vi "Init Control Value - Num.vi"(8 "error in (no error)":errorcluster, 10 "Num Control Names":string[](array[string]), 11 "This VI":refnum<vi>) -> (0 "error out":errorcluster, 2 "PLC IP":string, 3 "Config File Path":path)   [LabVIEW 2018]
uses:
  <vilib>/Utility/config.llb/Read Key (Double).vi
  <vilib>/Utility/config.llb/Write Key (Double).vi
  <vilib>/Utility/config.llb/Read Key (String).vi
  <vilib>/Utility/config.llb/NI_LVConfig.lvlib
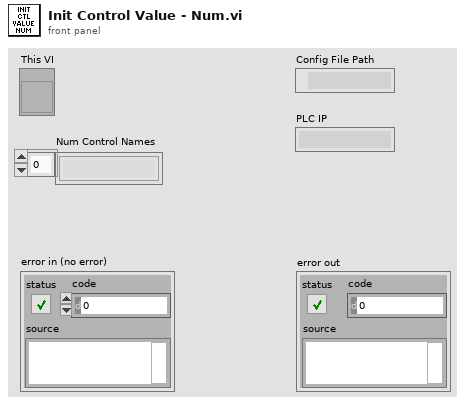
[diagram p1: front panel]
types:
  T1 = typedef "NI_LVConfig.lvlib/Config Data RefNum.ctl" = refnum<k1>
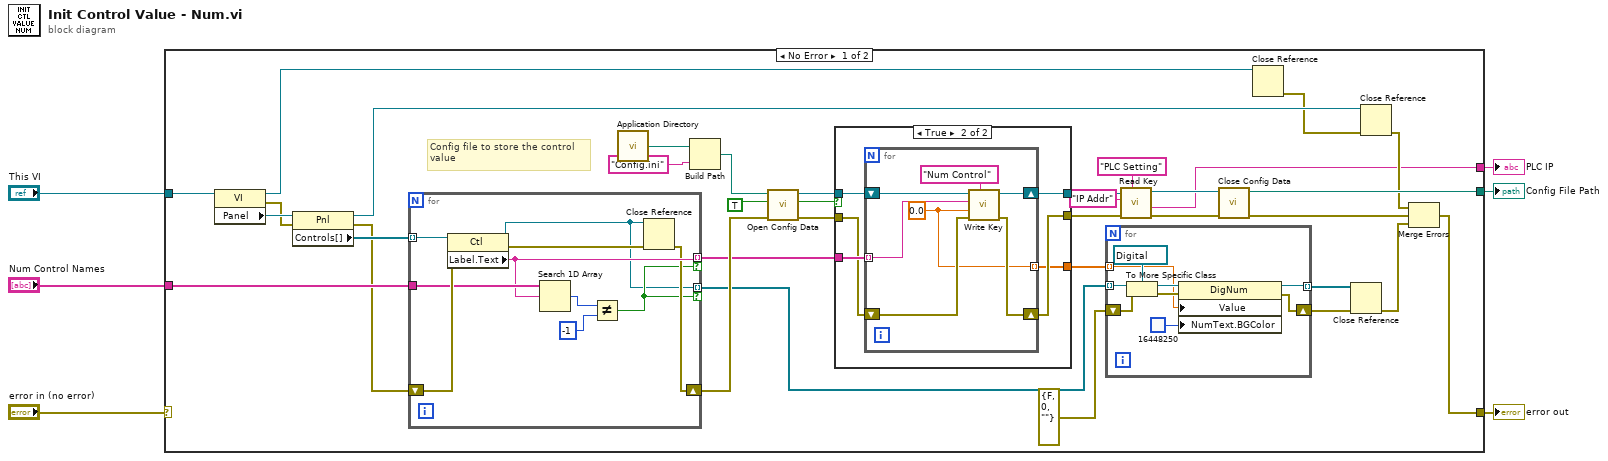
[diagram p0: block diagram]
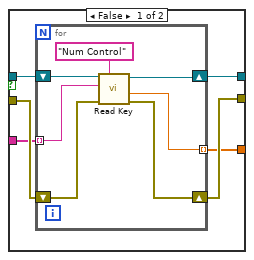
[diagram p2: hidden frame]
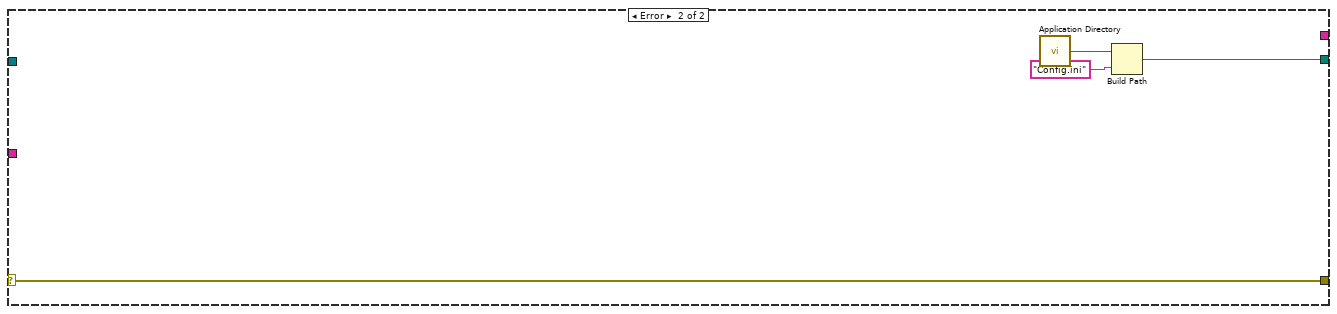
[diagram p3: hidden frame]
diagram:
  n1 = case shown="No Error" "error in (no error)" {
    selector: "error in (no error)" -> [_ w87]
    tunnel: "Num Control Names" -> [w38 _]
    tunnel: "This VI" -> [w39 _]
    tunnel: [w23 w88] -> w2
    tunnel: [w20 w87] -> w3
    tunnel: [w7 _] -> w1
    frame No Error {
      # "Config file to store the control\nvalue"
      n2 = property class="VI"(reference=w39) -> (reference out=w26:refnum<vi>, error out=w40:errorcluster, "Panel"=w41:refnum<vi>)  [unwired: 1 in]
      n3 = property class="Pnl"(reference=w41, error in=w40) -> (reference out=w25:refnum<vi>, error out=w36:errorcluster, "Controls[]"=w37:refnum<vi>[])
      n4 = for {
        tunnel: w37 -> [w86] mode=indexing
        shift-right: [w79] -> w34
        shift-left: w36 -> [w85]
        tunnel: w38 -> [w84]
        tunnel: [w81] -> w31 mode=indexing if=w78
        tunnel: [w77] -> w18 mode=indexing if=w78
        n5 = property class="Ctl"(reference=w86, error in=w85) -> (reference out=w77:refnum<vi>, error out=w80:errorcluster, "Label.Text"=w81:string)
        n6 = Search 1D Array(1D array=w84, element=w81) -> (index of element=w83:i32)  [unwired: 1 in]
        n7 = Not Equal?(x=w83, y=-1) -> (x != y?=w78:bool)
        n8 = Close Reference(reference=w77, error in (no error)=w80) -> (error out=w79:errorcluster)
      }
      n9 = call <vilib>:"Application Directory.vi"() -> ("Application Directory"=w29:path)
      n10 = Build Path(base path=w29, name or relative path="Config.ini") -> (appended path=w27:path)
      n11 = call <vilib>:"Open Config Data.vi"("error in (no error)"=w34, "create file if necessary (T)"=TRUE, "configuration file path"=w27) -> ("error out"=w30:errorcluster, "file created?"=w33:bool, "refnum"=w32:T1)  [unwired: 6 in]
      n12 = case shown="True" w33 {
        tunnel: w32 -> [w56 w68]
        tunnel: w31 -> [w54 w69]
        tunnel: w30 -> [w55 w67]
        tunnel: [w53 w66] -> w13
        tunnel: [w52 w65] -> w12
        tunnel: [w51 w64] -> w17
        frame False {
          n13 = for {
            shift-right: [w60] -> w53
            shift-left: w56 -> [w63]
            shift-right: [w58] -> w52
            shift-left: w55 -> [w61]
            tunnel: w54 -> [w59] mode=indexing
            tunnel: [w57] -> w51 mode=indexing
            n14 = call-poly <vilib>:"Read Key.vi"("section"="Num Control", "error in (no error)"=w61, "key"=w59, "refnum"=w63) -> ("error out"=w58:errorcluster, "value"=w57:dbl, "refnum out"=w60:T1)  [unwired: 4 in, 1 out]
          }
        }
        frame True {
          n15 = for {
            tunnel: w69 -> [w74] mode=indexing
            shift-right: [w72] -> w66
            shift-left: w68 -> [w75]
            shift-right: [w71] -> w65
            shift-left: w67 -> [w73]
            tunnel: [w70] -> w64 mode=indexing
            w70 = 0.0
            n16 = call-poly <vilib>:"Write Key.vi"("section"="Num Control", "error in (no error)"=w73, "value"=w70, "key"=w74, "refnum"=w75) -> ("error out"=w71:errorcluster, "refnum out"=w72:T1)  [unwired: 3 in, 2 out]
          }
        }
      }
      n17 = for {
        tunnel: w18 -> [w46] mode=indexing
        shift-right: [w43] -> w14
        shift-left: errorcluster {"status"=FALSE, "code"=0, "source"=""} ("error constant") -> [w45]
        tunnel: w17 -> [w44] mode=indexing
        tunnel: [w42] -> w16 mode=indexing
        n18 = To More Specific Class(target class=refnum<vi> refnum ("Numeric"), reference=w46, error in=w45) -> (specific class reference=w49:refnum<vi>, error out=w50:errorcluster)
        n19 = property class="DigNum"(reference=w49, error in=w50, "Value"=w44, "NumText.BGColor"=u32 16448250) -> (reference out=w42:refnum<vi>, error out=w43:errorcluster)
      }
      n20 = call-poly <vilib>:"Read Key.vi"("section"="PLC Setting", "error in (no error)"=w12, "key"="IP Addr", "refnum"=w13) -> ("error out"=w10:errorcluster, "value"=w7:string, "refnum out"=w11:T1)  [unwired: 4 in, 1 out]
      n21 = call <vilib>:"Close Config Data.vi"("error in (no error)"=w10, "refnum"=w11) -> ("error out"=w21:errorcluster, "file path"=w23:path)  [unwired: 8 in]
      n22 = Close Reference(reference=w26) -> (error out=w24:errorcluster)  [unwired: 1 in]
      n23 = Close Reference(reference=w16, error in (no error)=w14) -> (error out=w19:errorcluster)
      n24 = Close Reference(reference=w25, error in (no error)=w24) -> (error out=w22:errorcluster)
      n25 = Merge Errors(w22, w21, w19) -> (w20:errorcluster)
    }
    frame Error {
      n26 = call <vilib>:"Application Directory.vi"() -> ("Application Directory"=w90:path)
      n27 = Build Path(base path=w90, name or relative path="Config.ini") -> (appended path=w88:path)
    }
  }
  "error out" <- w3
  "Config File Path" <- w2
  "PLC IP" <- w1
